vi "Two button pneumatic.vi"(0 "Input 1":bool, 1 "Input 2":bool, 3 "State In":bool) -> (7 "Output 1":bool, 8 "Output 2":bool, 10 "State Out":bool)   [LabVIEW 2014]
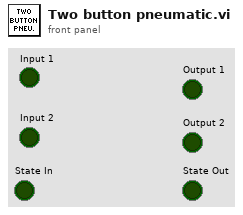
[diagram p1: front panel]
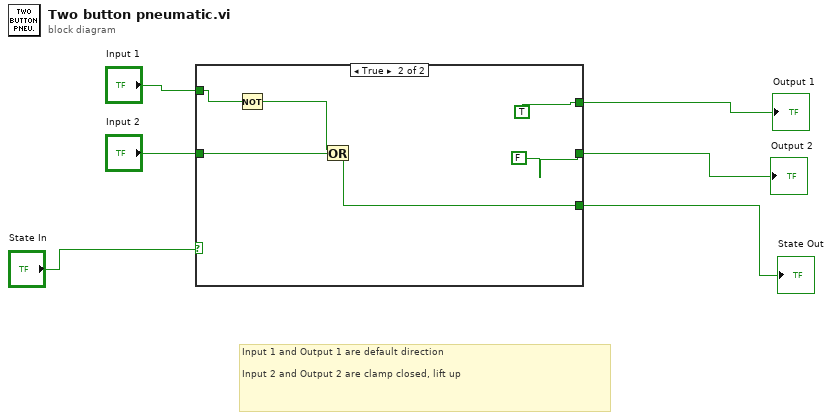
[diagram p0: block diagram]
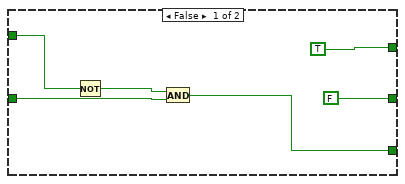
[diagram p2: hidden frame]
diagram:
  # "Input 1 and Output 1 are default direction\n\nInput 2 and Output 2 are clamp closed, lift up"
  n1 = case shown="True" "State In" {
    tunnel: "Input 1" -> [w12 w16]
    tunnel: "Input 2" -> [w10 w14]
    tunnel: [w9 w13] -> w3
    tunnel: [FALSE FALSE] -> w1
    tunnel: [TRUE TRUE] -> w2
    frame False {
      n2 = Not(x=w12) -> (.not. x?=w11:bool)
      n3 = And(x=w11, y=w10) -> (x .and. y?=w9:bool)
    }
    frame True {
      n4 = Not(x=w16) -> (.not. x?=w15:bool)
      n5 = Or(x=w15, y=w14) -> (x .or. y?=w13:bool)
    }
  }
  "Output 2" <- w1
  "State Out" <- w3
  "Output 1" <- w2
